vi "Del - UDP Data Link - Configuration Utilities - Set Tx Remove Channel Button.vi"(8 "error in (no error)":errorcluster, 11 "Tx ItemNames":string[][](array[string])) -> (0 "error out":errorcluster)   [LabVIEW 2015, in "UDP-Custom-Device System Explorer.lvlib"]
uses:
  UDP-Custom-Device System Explorer.lvlib
  Shared/Constants.vi
  <vilib>/NI VeriStand/Custom Device API/Custom Device API.lvlib
  Shared/UDP-Custom-Device Shared.lvlib
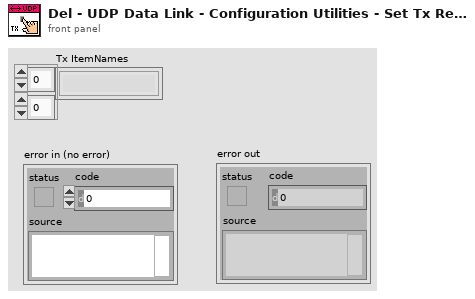
[diagram p1: front panel]
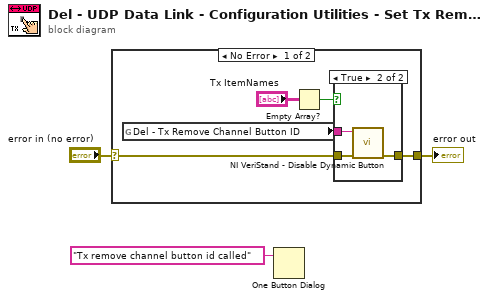
[diagram p0: block diagram]
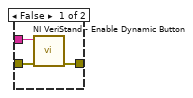
[diagram p2: hidden frame]
diagram:
  n1 = case shown="No Error" "error in (no error)" {
    selector: "error in (no error)" -> [w6 w15]
    tunnel: [w5 w15] -> w2
    frame No Error {
      n2 = global read "Constants.vi" "Del - Tx Remove Channel Button ID"() -> (w4:string)
      n3 = Empty Array?(array="Tx ItemNames") -> (empty?=w8:bool)
      n4 = case shown="True" w8 {
        tunnel: w4 -> [w11 w14]
        tunnel: w6 -> [w10 w13]
        tunnel: [w9 w12] -> w5
        frame False {
          n5 = call <vilib>:"NI VeriStand - Enable Dynamic Button.vi"("error in (no error)"=w10, "Button ID"=w11) -> ("error out"=w9:errorcluster)  [unwired: 9 in]
        }
        frame True {
          n6 = call <vilib>:"NI VeriStand - Disable Dynamic Button.vi"("error in (no error)"=w13, "Button ID"=w14) -> ("error out"=w12:errorcluster)  [unwired: 9 in]
        }
      }
    }
    frame Error {
    }
  }
  "error out" <- w2
  n7 = One Button Dialog(message="Tx remove channel button id called") -> ()  [unwired: 1 in, 1 out]
